vi "ImageAreaBackground.vi"(2 "Background":T1, 3 "Image":refnum<image>) -> (0 "Background Out":T1, 1 "OK Pressed":bool)   [LabVIEW 2009]
panel:
  in  "Background Color":u32(colorbox)
  in  "Fill Color":u32(colorbox)
  in  "Hatch Style":u32(ring) items=["Horizontal", "Vertical", "Forward Diagonal", "Backward Diagonal", "Cross", "Cross Hatch"]
  in  "Fill Style":u32(ring)=3 items=["Default"=3, "Solid"=0, "Hatch"=2]
  in  "Cancel Button":bool
  in  "OK Button":bool
  out "Preview":T2(plugin-control)
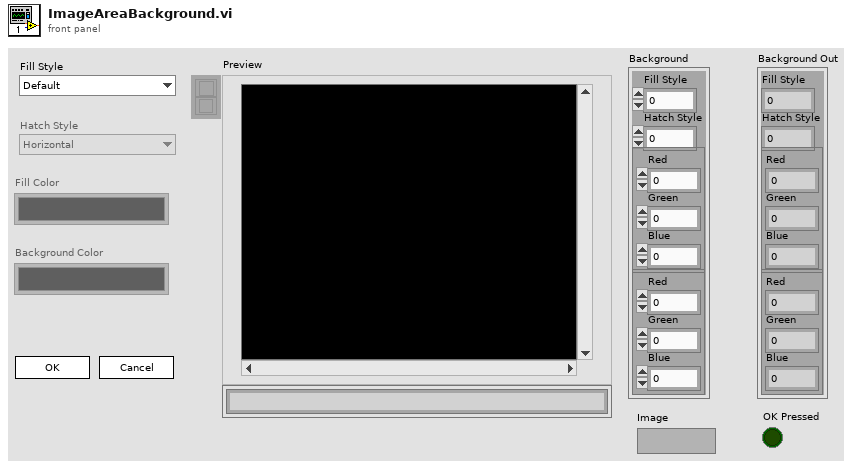
[diagram p1: front panel]
types:
  T1 = cluster{"Fill Style":u32, "Hatch Style":u32, cluster{"Red":u8, "Green":u8, "Blue":u8}, cluster{"Red":u8, "Green":u8, "Blue":u8}}
  T2 = typedef "IMAQ Image.ctl" = refnum<image>
  T3 = cluster{"Fill Style":u32, "Hatch Style":u32, "Fill Color":cluster{"Red":u8, "Green":u8, "Blue":u8}, "Background Color":cluster{"Red":u8, "Green":u8, "Blue":u8}}
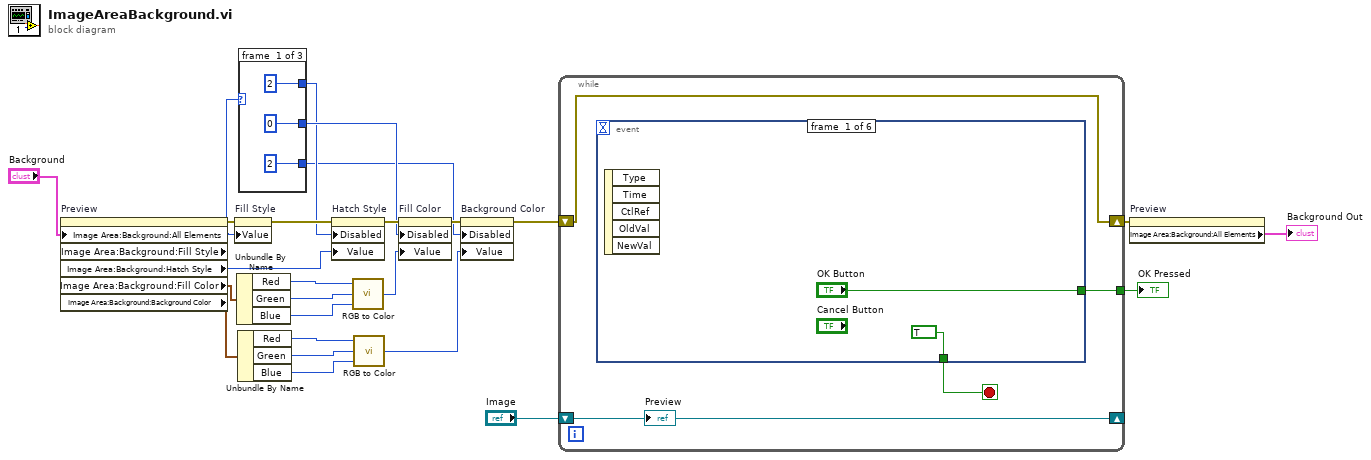
[diagram p0: block diagram]
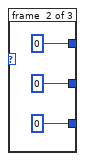
[diagram p2: hidden frame]
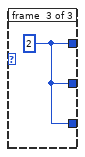
[diagram p3: hidden frame]
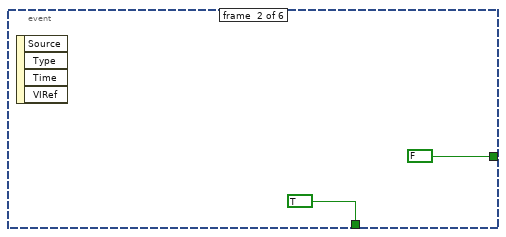
[diagram p4: hidden frame]
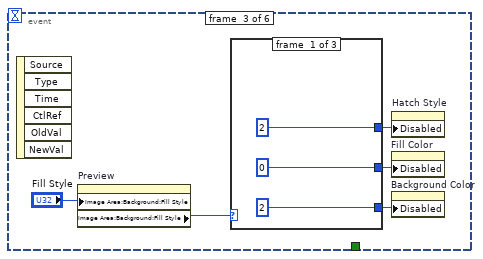
[diagram p5: hidden frame]
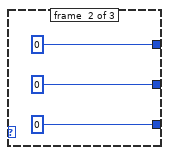
[diagram p6: hidden frame]
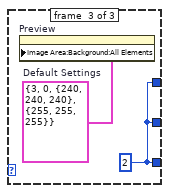
[diagram p7: hidden frame]
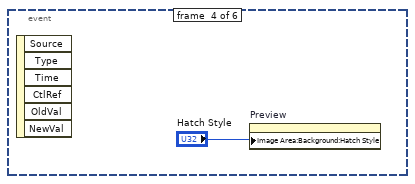
[diagram p8: hidden frame]
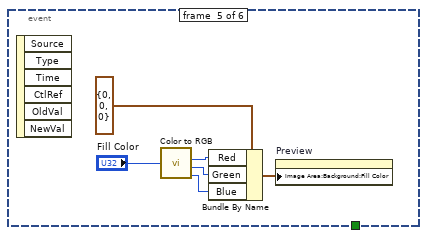
[diagram p9: hidden frame]
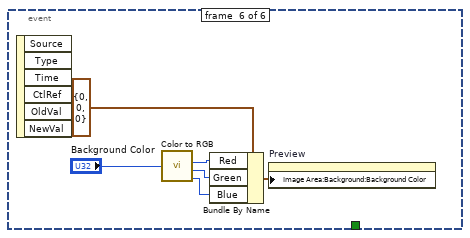
[diagram p10: hidden frame]
diagram:
  n1 = property on="Preview" class="ImageControl"("Image Area:Background:All Elements"="Background") -> (error out=w21:errorcluster, "Image Area:Background:Fill Style"=w8:u32, "Image Area:Background:Hatch Style"=w2:u32, "Image Area:Background:Fill Color"=w19:cluster{"Red":u8, "Green":u8, "Blue":u8}, "Image Area:Background:Background Color"=w11:cluster{"Red":u8, "Green":u8, "Blue":u8})  [unwired: 2 in, 1 out]
  n2 = property on="Fill Style" class="Ring (strict)"(error in=w21, "Value"=w8) -> (error out=w20:errorcluster)  [unwired: 1 in, 1 out]
  n3 = Unbundle By Name(w19) -> ("Red"=w18:u8, "Green"=w16:u8, "Blue"=w17:u8)
  n4 = Unbundle By Name(w11) -> ("Red"=w13:u8, "Green"=w15:u8, "Blue"=w14:u8)
  n5 = case shown="0" w8 {
    tunnel: [u8 2 ("Disabled") u8 0 ("Disabled") w32] -> w4
    tunnel: [u8 0 ("Disabled") u8 0 ("Disabled") w32] -> w5
    tunnel: [u8 2 ("Disabled") u8 0 ("Disabled") w32] -> w3
    frame #0 {
    }
    frame #1 {
    }
    frame #2 {
      w32 = u8 2 ("Disabled")
    }
  }
  n6 = property on="Hatch Style" class="Ring (strict)"(error in=w20, "Disabled"=w4, "Value"=w2) -> (error out=w12:errorcluster)  [unwired: 1 in, 1 out]
  n7 = call <vilib>:"RGB to Color.vi"("B"=w17, "G"=w16, "R"=w18) -> ("Color"=w6:u32)
  n8 = call <vilib>:"RGB to Color.vi"("B"=w14, "G"=w15, "R"=w13) -> ("Color"=w7:u32)
  n9 = property on="Fill Color" class="ColorBox"(error in=w12, "Disabled"=w5, "Value"=w6) -> (error out=w10:errorcluster)  [unwired: 1 in, 1 out]
  n10 = property on="Background Color" class="ColorBox"(error in=w10, "Disabled"=w3, "Value"=w7) -> (error out=w9:errorcluster)  [unwired: 1 in, 1 out]
  n11 = while {
    shift-right: [w35] -> w25
    shift-left: w9 -> [w35]
    shift-right: [w36] -> _
    shift-left: "Image" -> [w36]
    tunnel: [w33] -> w1
    stop <- w34 stop-if-true
    n12 = event shown="[2] \"Fill Style\": Value Change" {
      selector: _ -> [_ _ _ _ _ _]
      dyn-events: _ -> [_ _ _ _ _ _]
      timeout: _ -> [_ _ _ _ _ _]
      tunnel: [TRUE TRUE _ _ _ _] -> w34
      tunnel: ["OK Button" FALSE ("OK") _ _ _ _] -> w33
      event #0 {
        n13 = event-data() -> ()  [unwired: 1 in, 5 out]
      }
      event #1 {
        n14 = event-data() -> ()  [unwired: 1 in, 4 out]
      }
      event #2 {
        n15 = event-data() -> ()  [unwired: 1 in, 6 out]
        n16 = property on="Preview" class="ImageControl"("Image Area:Background:Fill Style"="Fill Style") -> ("Image Area:Background:Fill Style"=w44:u32)  [unwired: 2 in, 2 out]
        n17 = case shown="3, Default" w44 {
          tunnel: [u8 2 ("Disabled") u8 0 ("Disabled") w53] -> w43
          tunnel: [u8 0 ("Disabled") u8 0 ("Disabled") w53] -> w42
          tunnel: [u8 2 ("Disabled") u8 0 ("Disabled") w53] -> w41
          frame #0 {
          }
          frame #1 {
          }
          frame #2 {
            w52 = T3 {"Fill Style"=3, "Hatch Style"=0, "Fill Color"={"Red"=240, "Green"=240, "Blue"=240}, "Background Color"={"Red"=255, "Green"=255, "Blue"=255}}  # Default Settings
            w53 = u8 2 ("Disabled")
            n18 = property on="Preview" class="ImageControl"("Image Area:Background:All Elements"=w52) -> ()  [unwired: 2 in, 2 out]
          }
        }
        n19 = property on="Hatch Style" class="Ring (strict)"("Disabled"=w43) -> ()  [unwired: 2 in, 2 out]
        n20 = property on="Fill Color" class="ColorBox"("Disabled"=w42) -> ()  [unwired: 2 in, 2 out]
        n21 = property on="Background Color" class="ColorBox"("Disabled"=w41) -> ()  [unwired: 2 in, 2 out]
      }
      event #3 {
        n22 = event-data() -> ()  [unwired: 1 in, 6 out]
        n23 = property on="Preview" class="ImageControl"("Image Area:Background:Hatch Style"="Hatch Style") -> ()  [unwired: 2 in, 2 out]
      }
      event #4 {
        n24 = event-data() -> ()  [unwired: 1 in, 6 out]
        n25 = call <vilib>:"Color to RGB.vi"("Color"="Fill Color") -> ("R"=w58:u8, "G"=w59:u8, "B"=w60:u8)  [unwired: 1 out]
        n26 = Bundle By Name(cluster=cluster{"Red":u8, "Green":u8, "Blue":u8} {"Red"=0, "Green"=0, "Blue"=0} ("Image Area:Background:Background Color"), "Red"=w58, "Green"=w59, "Blue"=w60) -> (w55:cluster{"Red":u8, "Green":u8, "Blue":u8})
        n27 = property on="Preview" class="ImageControl"("Image Area:Background:Fill Color"=w55) -> ()  [unwired: 2 in, 2 out]
      }
      event #5 {
        n28 = event-data() -> ()  [unwired: 1 in, 6 out]
        n29 = call <vilib>:"Color to RGB.vi"("Color"="Background Color") -> ("R"=w64:u8, "G"=w63:u8, "B"=w62:u8)  [unwired: 1 out]
        n30 = Bundle By Name(cluster=cluster{"Red":u8, "Green":u8, "Blue":u8} {"Red"=0, "Green"=0, "Blue"=0} ("Image Area:Background:Background Color"), "Red"=w64, "Green"=w63, "Blue"=w62) -> (w61:cluster{"Red":u8, "Green":u8, "Blue":u8})
        n31 = property on="Preview" class="ImageControl"("Image Area:Background:Background Color"=w61) -> ()  [unwired: 2 in, 2 out]
      }
    }
    "Preview" <- w36
  }
  "OK Pressed" <- w1
  n32 = property on="Preview" class="ImageControl"(error in=w25) -> ("Image Area:Background:All Elements"=→"Background Out":T3)  [unwired: 1 in, 2 out]
